vi "myRIO__TCP_constants_byteRange_delim__checkRange.vi"(11 "input_byte":u8) -> (1 "output_delim_1":bool, 3 "output_delim":bool)   [LabVIEW 2014]
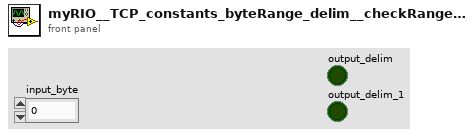
[diagram p1: front panel]
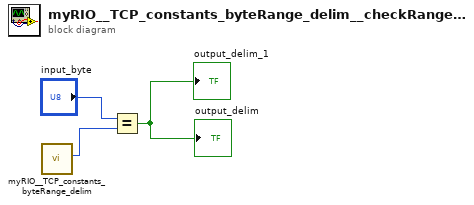
[diagram p0: block diagram]
diagram:
  n1 = call "myRIO__TCP_constants_byteRange_delim.vi"() -> ("output_delim_byte"=w3:u8)  [unwired: 10 in, 1 out]
  n2 = Equal?(x="input_byte", y=w3) -> (x = y?=→"output_delim" →"output_delim_1":bool)
